vi "session_set_additional_flag.vi"(6 "Skip setting if in Options string (F)":bool, 7 "AdditionalFlag Bit":T1, 8 "error in":errorcluster caption="error in (no error)", 10 "New value in":bool, 11 "VISA resource name":refnum<visa-resource-name>) -> (0 "error out":errorcluster, 2 "Old value out":bool, 3 "VISA resource name out":refnum<visa-resource-name>)   [LabVIEW 2022 SP3, in "hmp4000_rsidr_core.lvlib"]
doc: "OPC Timeout and VISA Timeout is not set if the 'int32 value in' is 0 or negative"
uses:
  hmp4000_rsidr_core.lvlib
  type_AdditionalFlag_Bits.ctl
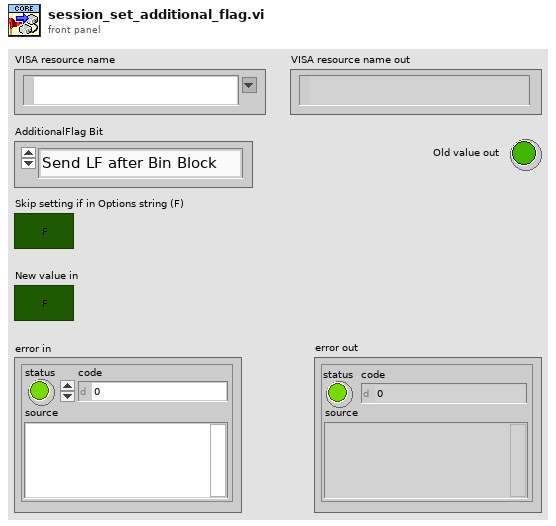
[diagram p1: front panel]
types:
  T1 = typedef "hmp4000_rsidr_core.lvlib/type_AdditionalFlag_Bits.ctl" = enum16{"Send LF after Bin Block", "Junk read with io_clear_buffers.vi", "io_clear_buffers: viClear()", "io_clear_buffers: viFlush()", "<NotUsed1>", "Allow Dbl & Int Bin/Ascii read", "*OPC? in check_instrument_error.vi", "<NotUsed2>", "Smart Enum Matching", "Less Strict RepCaps check", "AssureResponseEndWithLF"}
  T2 = typedef "hmp4000_rsidr_core.lvlib/type_Session_Data.ctl" = cluster{"IDN string":string, "Instrument FW":string, "Instr type":string, "Instr type for err. msg.":string, "Installed Options":string[], "Ignore Error Messages":string, "Logging params":variant, "OPC Timeout":i32, "VISA Timeout":i32, "STB Poll VISA Timeout":i32, "Additional Flags":i32, "Wait Before Read":i32, "Wait Before Write":i32, "Option String Flags":i32, "IO Segment Size":i64, "VISA Access Mode":T3, "Interface Type":T4, "OPC Wait Mode":T5, "Bin Float Number  Format":T6, "Bin Integer Number Format":T7, "Simulate":bool, "VXIcapable":bool, "Duplicate Session":bool, "Add LF to Write":bool, "Logging":bool, "Fast Sweep":bool, "Query Instrument Status":bool, "Check Range":bool, "Check Options":bool}
  T3 = typedef "hmp4000_rsidr_core.lvlib/type_VisaAccessMode.ctl" = u16
  T4 = typedef "hmp4000_rsidr_core.lvlib/type_InterfaceType.ctl" = enum16{"Unknown", "GPIB", "VXI", "GPIB_VXI", "ASRL", "PXI", "TCPIP", "USB", "SOCKET"}
  T5 = typedef "hmp4000_rsidr_core.lvlib/type_OPC_Wait_Mode.ctl" = enum16{"STBpolling", "STBpollingSlow", "STBpollingSuperSlow", "ServiceRequest", "OPCquery"}
  T6 = typedef "hmp4000_rsidr_core.lvlib/type_Binary_Float_Number_Format.ctl" = enum16{"Float_4_Bytes_Swapped", "Float_4_Bytes", "Double_8_Bytes_Swapped", "Double_8_Bytes"}
  T7 = typedef "hmp4000_rsidr_core.lvlib/type_Binary_Integer_Number_Format.ctl" = enum16{"Int32_4_Bytes_Swapped", "Int32_4 Bytes", "Int16_2_Bytes_Swapped", "Int16_2_Bytes"}
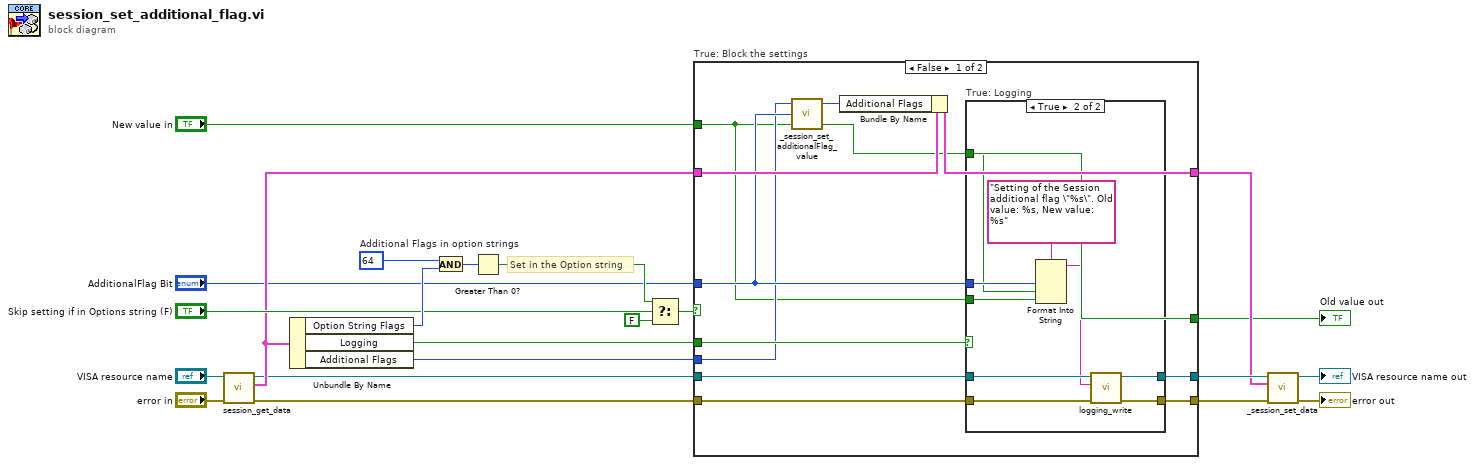
[diagram p0: block diagram]
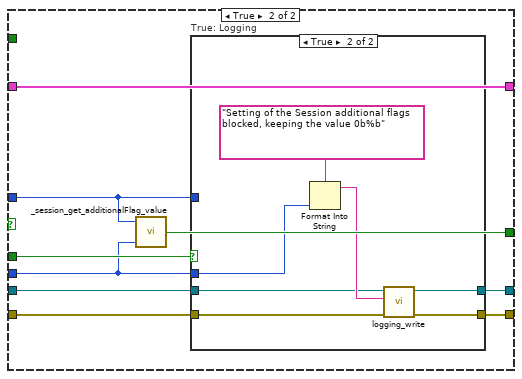
[diagram p3: hidden frame]
diagram:
  w7 = 64  # Additional Flags in option strings
  # "Set in the Option string"
  n1 = call "session_get_data.vi"("error in"="error in", "VISA resource name"="VISA resource name") -> ("error out"=w5:errorcluster, "Session User Data out"=w9:T2, "VISA resource name out"=w4:refnum<visa-resource-name>)  [unwired: 6 in, 1 out]
  n2 = Unbundle By Name(w9) -> ("Option String Flags"=w14:i32, "Logging"=w13:bool, "Additional Flags"=w3:i32)
  n3 = And(x=w7, y=w14) -> (x .and. y?=w22:i32)
  n4 = Greater Than 0?(x=w22) -> (x > 0?=w11:bool)
  n5 = Select(t=w11, s="Skip setting if in Options string (F)", f=FALSE) -> (s? t:f=w6:bool)
  n6 = case "True: Block the settings" shown="False" w6 {
    tunnel: "AdditionalFlag Bit" -> [w27 w48]
    tunnel: w9 -> [w34 w49]
    tunnel: "New value in" -> [w23 _]
    tunnel: [w33 w49] -> w15
    tunnel: w5 -> [w32 w53]
    tunnel: w4 -> [w31 w52]
    tunnel: [w30 w51] -> w19
    tunnel: [w29 w50] -> w18
    tunnel: w13 -> [w28 w54]
    tunnel: w3 -> [w26 w46]
    tunnel: [w24 w47] -> w1
    frame False {
      n7 = call "_session_set_additionalFlag_value.vi"("New value in"=w23, "AdditionalFlag bit"=w27, "Additional Flags in"=w26) -> ("Old value out"=w24:bool, "Additional Flags out"=w25:i32)  [unwired: 1 in]
      n8 = Bundle By Name(cluster=w34, "Additional Flags"=w25) -> (w33:T2)
      n9 = case "True: Logging" shown="True" w28 {
        tunnel: w27 -> [_ w40]
        tunnel: w32 -> [w35 w44]
        tunnel: w31 -> [w36 w43]
        tunnel: [w35 w42] -> w30
        tunnel: [w36 w41] -> w29
        tunnel: w23 -> [_ w38]
        tunnel: w24 -> [_ w39]
        frame False {
        }
        frame True {
          n10 = Format Into String(format string="Setting of the Session additional flag \"%s\". Old value: %s, New value: %s", w40, w39, w38) -> (resulting string=w37:string)  [unwired: 2 in, 1 out]
          n11 = call "logging_write.vi"("error in"=w44, "String to write"=w37, "VISA resource name"=w43) -> ("error out"=w42:errorcluster, "VISA resource name out"=w41:refnum<visa-resource-name>)  [unwired: 7 in]
        }
      }
    }
    frame True {
      n12 = call "_session_get_additionalFlag_value.vi"("AdditionalFlags value in"=w46, "AdditionalFlag bit"=w48) -> ("AdditionalFlag bit value out"=w47:bool)  [unwired: 3 in]
      n13 = case "True: Logging" shown="True" w54 {
        tunnel: w53 -> [w56 w61]
        tunnel: w52 -> [w55 w60]
        tunnel: [w56 w59] -> w51
        tunnel: [w55 w58] -> w50
        tunnel: w48 -> [_ _]
        tunnel: w46 -> [_ w57]
        frame False {
        }
        frame True {
          n14 = Format Into String(format string="Setting of the Session additional flags blocked, keeping the value 0b%b", w57) -> (resulting string=w62:string)  [unwired: 2 in, 1 out]
          n15 = call "logging_write.vi"("error in"=w61, "String to write"=w62, "VISA resource name"=w60) -> ("error out"=w59:errorcluster, "VISA resource name out"=w58:refnum<visa-resource-name>)  [unwired: 7 in]
        }
      }
    }
  }
  "Old value out" <- w1
  n16 = call "_session_set_data.vi"("error in"=w19, "Session User Data in"=w15, "VISA resource name"=w18) -> ("error out"=→"error out":errorcluster, "VISA resource name out"=→"VISA resource name out":refnum<visa-resource-name>)  [unwired: 7 in]
